vi "UserDefined.Group.Export.vi"(8 "error in (no error)":errorcluster, 11 "Item Ref in":T1 format="%.0x") -> (0 "error out":errorcluster, 2 "Group":T2 {"Messages"."Signals"."Response"."Byte Order" items=["Little Endian", "Big Endian"]; "Messages"."Signals"."Response"."Data Type" items=["Signed", "Unsigned", "IEEE Float"]; "Messages"."Signals"."Cmd"."Byte Order" items=["Little Endian", "Big Endian"]; "Messages"."Signals"."Cmd"."Data Type" items=["Signed", "Unsigned", "IEEE Float"]}, 3 "Section Ref out":T1 format="%.0x")   [LabVIEW 2015, in "Diagnostics Addon System Explorer.lvlib"]
uses:
  Diagnostics Addon System Explorer.lvlib
  <vilib>/NI Veristand/Custom Device API/Custom Device Item Ref.ctl
  Types/UserDefined.Group.Export.ctl
  Types/UserDefined.Group.Message.Export.ctl
  Types/CmdResp.Export.ctl
  Shared/Types/Signal.ctl
  Signals.Get.vi
  Type.FG.vi
  Signal.FG.vi
  <vilib>/NI Veristand/Custom Device API/NI VeriStand - Get Item Property.vi
  <vilib>/NI Veristand/Custom Device API/Get Item Property (U32).vi
  <vilib>/NI/NIVS System Definition Utilities/SysDef API/SysDef.Property.Set.vi
  <vilib>/NI/NIVS System Definition Utilities/_SubVIs/SysDef.Property.Set.U32.vi
  Shared/SubVIs/Constants.vi
  <vilib>/NI Veristand/Custom Device API/NI VeriStand - Get Custom Device Channel Data.vi
  <vilib>/NI Veristand/Custom Device API/Get Item Property (String).vi
  <vilib>/NI Veristand/Custom Device API/Get Item Property (Double).vi
  <vilib>/NI/NIVS System Definition Utilities/_SubVIs/SysDef.Property.Set.String.vi
  <vilib>/NI/NIVS System Definition Utilities/_SubVIs/SysDef.Property.Set.DBL.vi
  <vilib>/NI Veristand/Custom Device API/NI VeriStand - Get Item Children.vi
  <vilib>/NI Veristand/Custom Device Tools/Custom Device Utility Library/NI VeriStand - Search for Item by GUID.vi
  <vilib>/NI Veristand/Custom Device Tools/Custom Device Utility Library/NI VeriStand - Search for All Items by GUID.vi
  Shared/Diagnostics Addon Shared.lvlib
  <vilib>/NI VeriStand/Custom Device API/Custom Device API.lvlib
  <vilib>/NI Veristand/Custom Device Tools/Custom Device Utility Library/Custom Device Utility Library.lvlib
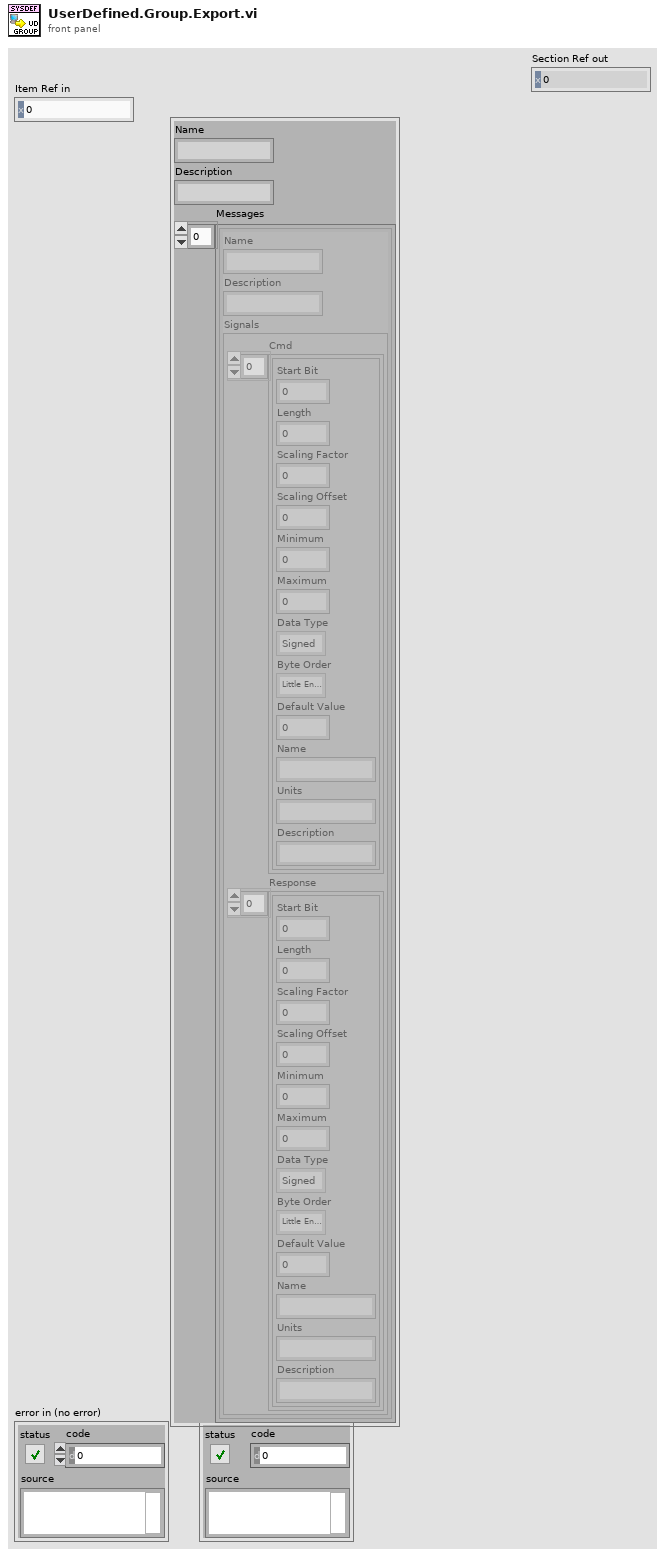
[diagram p1: front panel]
types:
  T1 = typedef "Custom Device API.lvlib/Custom Device Item Ref.ctl" = u64
  T2 = typedef "Diagnostics Addon System Explorer.lvlib/UserDefined.Group.Export.ctl" = cluster{"Name":string, "Description":string, "Messages":T3[]}
  T3 = typedef "Diagnostics Addon System Explorer.lvlib/UserDefined.Group.Message.Export.ctl" = cluster{"Name":string, "Description":string, "Signals":T4}
  T4 = typedef "Diagnostics Addon System Explorer.lvlib/CmdResp.Export.ctl" = cluster{"Cmd":T5[], "Response":T5[]}
  T5 = typedef "Diagnostics Addon Shared.lvlib/Signal.ctl" = cluster{"Start Bit":u32, "Length":u32, "Scaling Factor":dbl, "Scaling Offset":dbl, "Minimum":dbl, "Maximum":dbl, "Data Type":u32, "Byte Order":u32, "Default Value":dbl, "Name":string, "Units":string, "Description":string}
  T6 = typedef "Custom Device API.lvlib/Custom Device Item Info.ctl" = cluster{"Name":string, "Is Channel":bool, "GUID":string, "Is Waveform":bool}
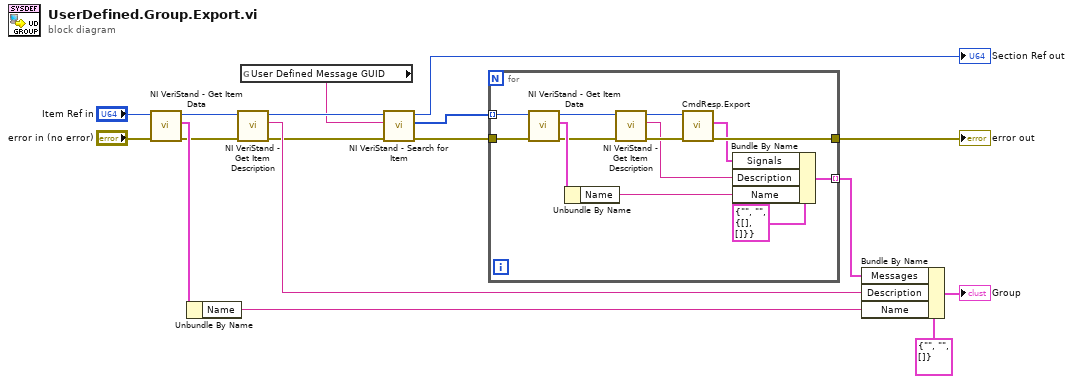
[diagram p0: block diagram]
diagram:
  n1 = call <vilib>:"NI VeriStand - Get Item Data.vi"("error in (no error)"="error in (no error)", "Item Ref in"="Item Ref in") -> ("error out"=w15:errorcluster, "Item Info"=w16:T6, "Item Ref out"=w13:T1)  [unwired: 6 in, 1 out]
  n2 = Unbundle By Name(w16) -> ("Name"=w8:string)
  n3 = call <vilib>:"NI VeriStand - Get Item Description.vi"("error in (no error)"=w15, "Item Ref in"=w13) -> ("error out"=w3:errorcluster, "Description"=w11:string, "Item Ref out"=w6:T1)  [unwired: 6 in, 1 out]
  n4 = global read "Constants.vi" "User Defined Message GUID"() -> (w4:string)
  n5 = call-poly <vilib>:"NI VeriStand - Search for Item.vi"("error in"=w3, "Item GUID"=w4, "Section Ref in"=w6) -> ("error out"=w2:errorcluster, "Item Refs"=w5:T1[], "Section Ref out"=→"Section Ref out":T1)  [unwired: 5 in, 1 out]
  n6 = for {
    tunnel: [w30] -> w17
    tunnel: [w18] -> w9 mode=indexing
    tunnel: w5 -> [w26] mode=indexing
    tunnel: w2 -> [w25]
    n7 = call <vilib>:"NI VeriStand - Get Item Data.vi"("error in (no error)"=w25, "Item Ref in"=w26) -> ("error out"=w28:errorcluster, "Item Info"=w29:T6, "Item Ref out"=w27:T1)  [unwired: 6 in, 1 out]
    n8 = Unbundle By Name(w29) -> ("Name"=w21:string)
    n9 = call <vilib>:"NI VeriStand - Get Item Description.vi"("error in (no error)"=w28, "Item Ref in"=w27) -> ("error out"=w24:errorcluster, "Description"=w20:string, "Item Ref out"=w23:T1)  [unwired: 6 in, 1 out]
    n10 = call "CmdResp.Export.vi"("error in (no error)"=w24, "Device Item Ref in"=w23) -> ("error out"=w30:errorcluster, "Signals"=w19:T4)  [unwired: 7 in, 1 out]
    n11 = Bundle By Name(cluster=T3 {"Name"="", "Description"="", "Signals"={"Cmd"=[], "Response"=[]}} ("IO Control"), "Signals"=w19, "Description"=w20, "Name"=w21) -> (w18:T3)
  }
  "error out" <- w17
  n12 = Bundle By Name(cluster=T2 {"Name"="", "Description"="", "Messages"=[]} ("IO"), "Messages"=w9, "Description"=w11, "Name"=w8) -> (→"Group":T2)
